vi "cycle select all requested.vi"(7 "which value to be selected":T2, 8 "error in":errorcluster, 9 "value that will be sorted In":i32, 11 "cycle results cluster IN":T1) -> (0 "error out":errorcluster, 3 "cycle results cluster out":T1 {"cycle results dbl" format="%#_6e"})   [LabVIEW 2016]
doc: "Takes the desired value for the selected array and pulls out only the specific cycles"
uses:
  controls/cycle results control.ctl
  controls/unique results control.ctl
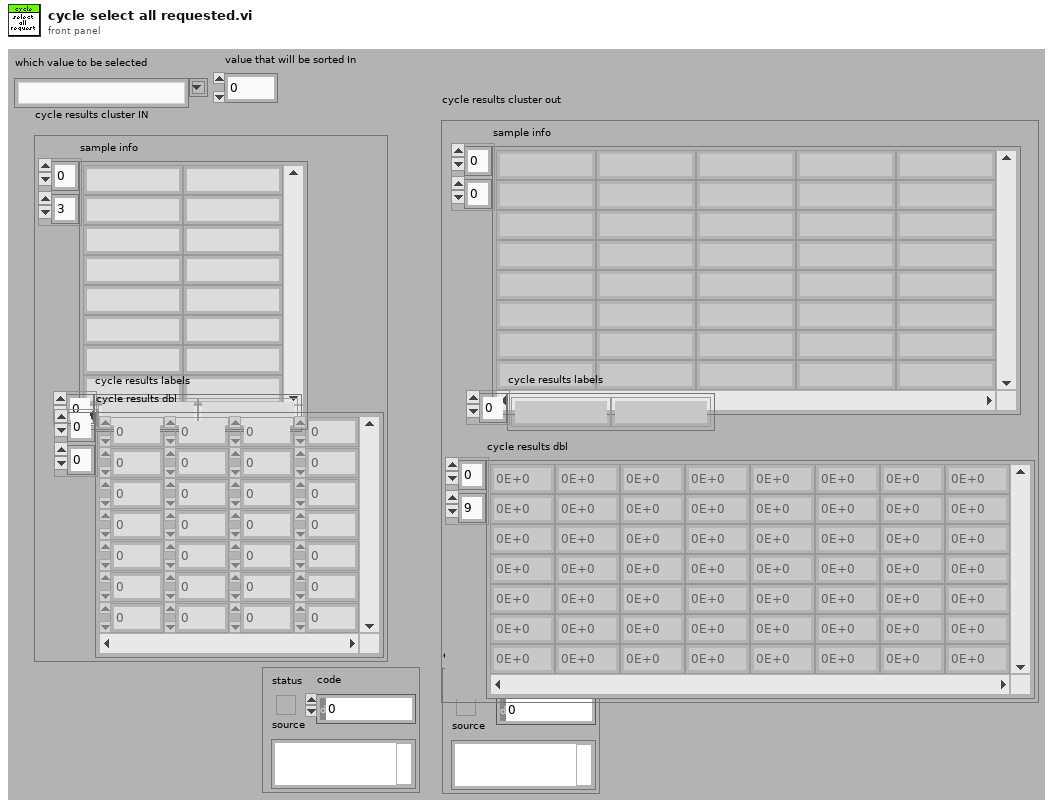
[diagram p1: front panel]
types:
  T1 = typedef "cycle results control.ctl" = cluster{"sample info":string[][], "cycle results labels":string[], "cycle results dbl":dbl[][]}
  T2 = typedef "unique results control.ctl" = string
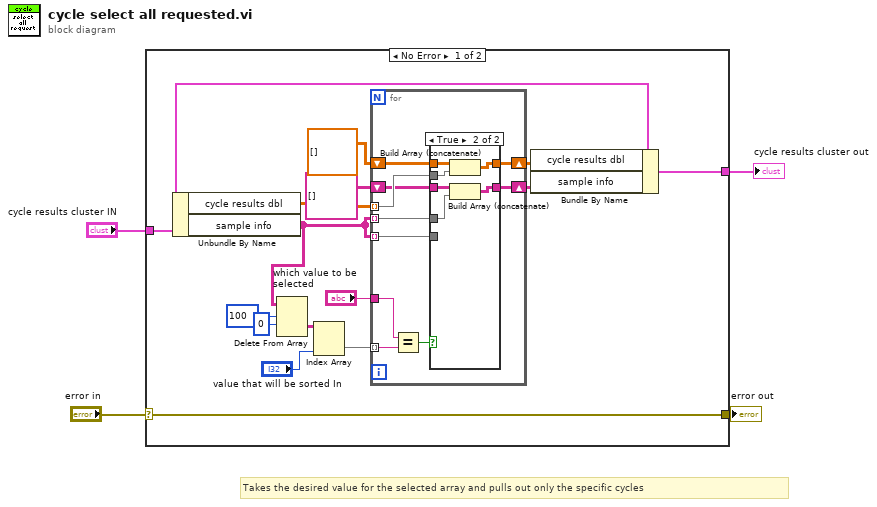
[diagram p0: block diagram]
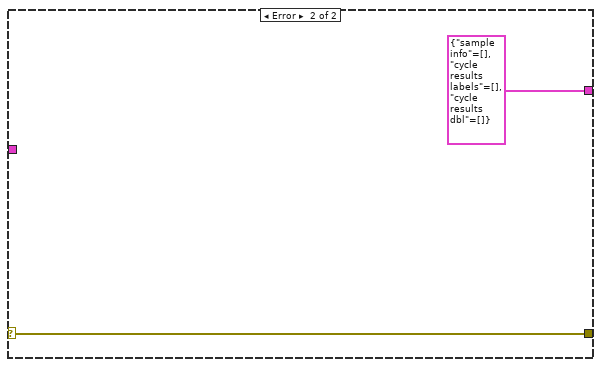
[diagram p3: hidden frame]
diagram:
  # "Takes the desired value for the selected array and pulls out only the specific cycles"
  n1 = case shown="No Error" "error in" {
    selector: "error in" -> [w11 w39]
    tunnel: "cycle results cluster IN" -> [w14 _]
    tunnel: [w12 T1 {"sample info"=[], "cycle results labels"=[], "cycle results dbl"=[]} ("cycle results cluster IN")] -> w3
    tunnel: [w11 w39] -> w1
    frame No Error {
      n2 = Unbundle By Name(w14) -> ("cycle results dbl"=w17:dbl[][], "sample info"=w8:string[][])
      n3 = Delete From Array(array=w8, length=100, index (row)=0) -> (deleted portion=w5:string[][])  [unwired: 1 in, 1 out]
      n4 = Index Array(array=w5, index (col)="value that will be sorted In") -> (element=w19:string[])  [unwired: 1 in]
      n5 = for {
        tunnel: w19 -> [w29] mode=indexing
        tunnel: "which value to be selected" -> [w28]
        tunnel: w17 -> [w26] mode=indexing
        shift-right: [w25] -> w15
        shift-left: dbl[][] [] -> [w24]
        tunnel: w8 -> [w23] mode=indexing
        tunnel: w8 -> [w22] mode=indexing
        shift-right: [w21] -> w10
        shift-left: string[][] [] -> [w20]
        n6 = Equal?(x=w28, y=w29) -> (x = y?=w27:bool)
        n7 = case shown="True" w27 {
          tunnel: w26 -> [_ w37]
          tunnel: [w31 w36] -> w25
          tunnel: w24 -> [w31 w35]
          tunnel: w23 -> [_ _]
          tunnel: w22 -> [_ w34]
          tunnel: [w30 w33] -> w21
          tunnel: w20 -> [w30 w32]
          frame False {
          }
          frame True {
            n8 = Build Array (concatenate)(w35, w37) -> (w36:dbl[][])
            n9 = Build Array (concatenate)(w32, w34) -> (w33:string[][])
          }
        }
      }
      n10 = Bundle By Name(cluster=w14, "cycle results dbl"=w15, "sample info"=w10) -> (w12:T1)
    }
    frame Error {
    }
  }
  "error out" <- w1
  "cycle results cluster out" <- w3
